vi "read_OSC.vi"(8 "error in (no error)":errorcluster, 10 "Channel (0: Channel 1)":u16(ring)=1 items=["Channel 1", "Channel 2", "Channel 3", "Channel 4", "Math 1", "Math 2", "Math 3", "Math 4", "Reference 1", "Reference 2", "Reference 3", "Reference 4"]) -> (0 "error out":errorcluster, 3 "VISA resource name out":refnum<visa-resource-name>, 4 "appended array":dbl[][][](array[numeric]), 5 "dt":dbl)   [LabVIEW 2011]
doc: "Triggers measurement and reads the waveform data from the OSC. \nThe fast frame-frames are split up into background (BG) and molecular (mol.) frames. The output array consists of the following parts:\n- av. bg frames \n- raw bg frames (with n-sub arrays)\n- av. mol frames \n- raw mol frames (with n-sub arrays)"
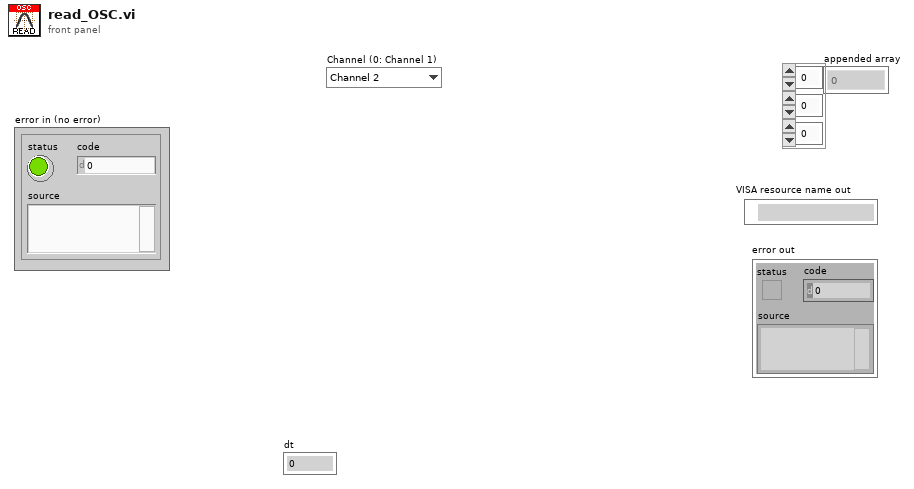
[diagram p1: front panel]
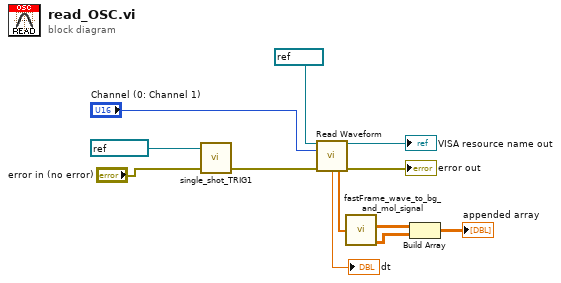
[diagram p0: block diagram]
diagram:
  n1 = call "single_shot_TRIG1.vi"("error in (no error)"="error in (no error)", "VISA resource name"=refnum<visa-resource-name> "TRIG1") -> ("error out"=w11:errorcluster)  [unwired: 2 in, 1 out]
  n2 = call "Read Waveform.vi"("VISA resource name"=refnum<visa-resource-name> "OSC", "Channel (0: Channel 1)"="Channel (0: Channel 1)", "error in (no error)"=w11) -> ("VISA resource name out"=→"VISA resource name out":refnum<visa-resource-name>, "dt"=→"dt":dbl, "raw array data"=w10:dbl[], "error out"=→"error out":errorcluster)  [unwired: 8 in, 1 out]
  n3 = call "fastFrame_wave_to_bg_and_mol_signal.vi"("all fast frames"=w10) -> ("bg frames"=w3:dbl[][], "mol. frames"=w2:dbl[][])  [unwired: 4 in]
  n4 = Build Array(w3, w2) -> (→"appended array":dbl[][][])
